vi "JSONtext Pretty Print.vi"(11 "JSON":string) -> (2 "Value String":string, 3 "Boolean":bool)   [LabVIEW 2019]
uses:
  JDP Science/JSONtext/JSONtext.lvlib
panel:
  out "String":string
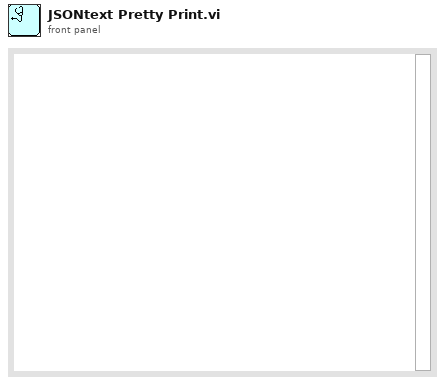
[diagram p1: front panel]
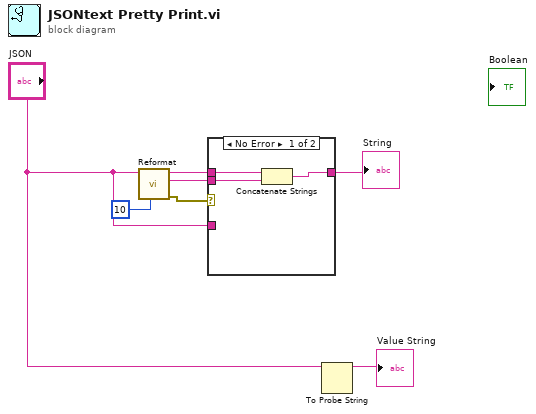
[diagram p0: block diagram]
diagram:
  n1 = call "Reformat.vi"("Pretty Print Levels"=10, "JSON"="JSON") -> ("error out"=w6:errorcluster, "Rest of Input String"=w1:string, "<JSON>"=w5:string)  [unwired: 6 in, 1 out]
  n2 = case shown="No Error" w6 {
    tunnel: [w9 w11] -> w4
    tunnel: w5 -> [w10 _]
    tunnel: "JSON" -> [_ w11]
    tunnel: w1 -> [w8 _]
    frame No Error {
      n3 = Concatenate Strings(w10, w8) -> (w9:string)
    }
    frame Error {
    }
  }
  "String" <- w4
  n4 = To Probe String(7:"JSON") -> (3:→"Value String":string)  [unwired: 2 in, 1 out]
